vi "例4-22.vi"   [LabVIEW 2019]
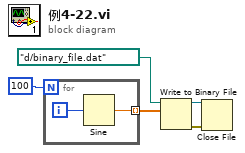
[diagram p0: block diagram]
diagram:
  n1 = for {
    N: 100 -> [_]
    tunnel: [w6] -> w1 mode=indexing
    i -> [w7]
    n2 = Sine(x=w7) -> (sin(x)=w6:dbl)
  }
  n3 = Write to Binary File(file (use dialog)=path "d:/binary_file.dat" ("文件（使用对话框）"), data=w1) -> (refnum out=w3:refnum<file>, error out=w4:errorcluster)  [unwired: 4 in, 1 out]
  n4 = Close File(refnum=w3, error in=w4) -> ()  [unwired: 2 out]
